vi "Agilent N6900 N7900 Series Output Current List.vi"() -> ()   [LabVIEW 2021]
doc: "This example demonstrates how to configure a list in current priority mode."
uses:
  <instrlib>/Agilent N6900 N7900 Series/Agilent N6900 N7900 Series.lvlib
panel:
  in  "Dwell Points":dbl[](array[numeric])
  in  "Current Points":dbl[](array[numeric])
  in  "Current Priority Voltage Limit (25V)":dbl=25.0
  in  "VISA resource name":refnum<visa-resource-name>
  # "(c) 2013-2018 National Instruments Corporation.  ALL RIGHTS RESERVED."
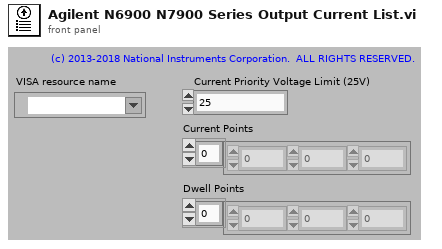
[diagram p1: front panel]
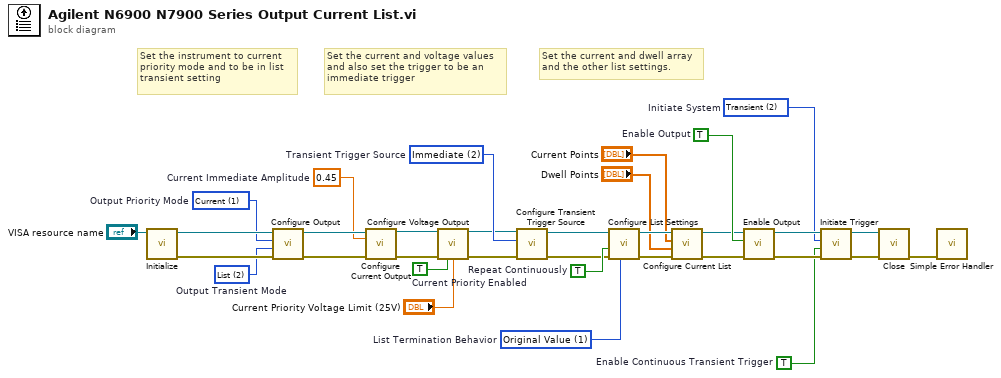
[diagram p0: block diagram]
diagram:
  w13 = TRUE  # Enable Output
  w14 = TRUE  # Enable Continuous Transient Trigger
  w15 = u16 2 items=["Acquisition", "External Logging", "Transient"]  # Initiate System
  w16 = u16 2 items=["Bus", "External", "Immediate", "Pin 1", "Pin 2", "Pin 3", "Pin 4", "Pin 5", "Pin 6", "Pin 7"]  # Transient Trigger Source
  w24 = u16 1 items=["Last Value", "Original Value"]  # List Termination Behavior
  w25 = TRUE  # Repeat Continuously
  w8 = TRUE  # Current Priority Enabled
  w27 = 0.45  # Current Immediate Amplitude
  w30 = u16 2 items=["Fixed", "Step", "List", "Arbitrary"]  # Output Transient Mode
  w31 = u16 1 items=["Voltage", "Current"]  # Output Priority Mode
  # "Set the current and dwell array\nand the other list settings."
  # "Set the current and voltage values\nand also set the trigger to be an\nimmediate trigger"
  # "Set the instrument to current \npriority mode and to be in list\ntransient setting"
  n1 = call <instrlib>:"Initialize.vi"("VISA resource name"="VISA resource name") -> ("error out"=w32:errorcluster, "VISA resource name out"=w33:refnum<visa-resource-name>)  [unwired: 9 in]
  n2 = call <instrlib>:"Configure Output.vi"("error in (no error)"=w32, "Output Transient Mode (0: Fixed)"=w30, "Output Priority Mode (0: Voltage)"=w31, "VISA resource name"=w33) -> ("error out"=w28:errorcluster, "VISA resource name out"=w29:refnum<visa-resource-name>)  [unwired: 6 in]
  n3 = call <instrlib>:"Configure Current Output.vi"("VISA resource name"=w29, "Current Immediate Amplitude (0 A)"=w27, "error in (no error)"=w28) -> ("VISA resource name out"=w9:refnum<visa-resource-name>, "error out"=w12:errorcluster)  [unwired: 11 in]
  n4 = call <instrlib>:"Configure Voltage Output.vi"("VISA resource name"=w9, "error in (no error)"=w12, "Enable Current Priority (False)"=w8, "Current Priority Voltage Limit (25V)"="Current Priority Voltage Limit (25V)") -> ("VISA resource name out"=w10:refnum<visa-resource-name>, "error out"=w11:errorcluster)  [unwired: 10 in]
  n5 = call <instrlib>:"Configure Transient Trigger Source.vi"("error in (no error)"=w11, "Transient Trigger Source (0: Bus)"=w16, "VISA resource name"=w10) -> ("error out"=w18:errorcluster, "VISA resource name out"=w17:refnum<visa-resource-name>)  [unwired: 7 in]
  n6 = call <instrlib>:"Configure List Settings.vi"("List Termination Behavior (1: Last Value)"=w24, "error in (no error)"=w18, "Repeat Continuously (False)"=w25, "VISA resource name"=w17) -> ("error out"=w3:errorcluster, "VISA resource name out"=w4:refnum<visa-resource-name>)  [unwired: 6 in]
  n7 = call <instrlib>:"Configure Current List.vi"("error in (no error)"=w3, "Dwell Points"="Dwell Points", "Current Points"="Current Points", "VISA resource name"=w4) -> ("error out"=w6:errorcluster, "VISA resource name out"=w5:refnum<visa-resource-name>)  [unwired: 6 in]
  n8 = call <instrlib>:"Enable Output.vi"("error in (no error)"=w6, "Enable Output (F: Disable)"=w13, "VISA resource name"=w5) -> ("error out"=w22:errorcluster, "VISA resource name out"=w23:refnum<visa-resource-name>)  [unwired: 7 in]
  n9 = call <instrlib>:"Initiate Trigger.vi"("error in (no error)"=w22, "Enable Continuous Transient Trigger (T: Enable)"=w14, "Initiate System (0: Acquisition)"=w15, "VISA resource name"=w23) -> ("error out"=w20:errorcluster, "VISA resource name out"=w21:refnum<visa-resource-name>)  [unwired: 6 in]
  n10 = call <instrlib>:"Close.vi"("error in (no error)"=w20, "VISA resource name"=w21) -> ("error out"=w19:errorcluster)  [unwired: 9 in]
  n11 = call <vilib>:"Simple Error Handler.vi"("error in (no error)"=w19) -> ()  [unwired: 4 in, 5 out]
